vi "Prefilter.60Hz_Notch.vi"(8 "error in (no error)":errorcluster, 11 "Instrument.DAQ":refnum<class "Instrument.DAQ.lvclass">) -> (0 "error out":errorcluster, 3 "Instrument.DAQ out":refnum<class "Instrument.DAQ.lvclass">)   [LabVIEW 2019, in "Instrument.Lockin.lvlib" / "Instrument.DAQ.lvclass"]
uses:
  Instrument.DAQ.lvclass
  Instrument.DAQ.lvclass/Instrument.DAQ.ctl
  <vilib>/addons/Digital Filter Design/Design.llb/DFD IIR Notch Peak Design by Q.vi
  <vilib>/addons/Digital Filter Design/NI_DigFilterLicensed.lvlib
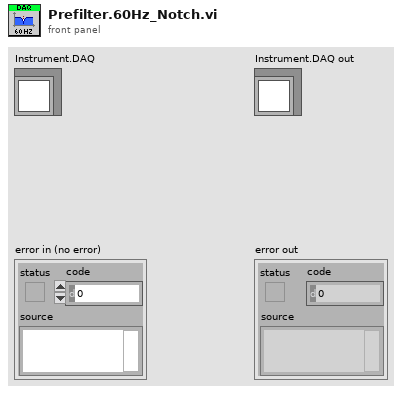
[diagram p1: front panel]
types:
  T1 = typedef "NI_DigFilterLicensed.lvlib/DFD Filter Obj.ctl" = cluster{"mSRate_Fs":dbl, "mSRate_Version":string, "mSRate_Comments":string, "mSRate_OrgCoef":T2, "mSRate_CurCoef":T2, "mSRate_Quantized?":bool, "mSRate_QCoef":T2, "mSRate_QSettings":T4[], "mSRate_Order":i32, "mSRate_Scaling":cluster{"mSRate_ScaleByPowerOf2?":bool, "mSRate_ScaleType":T6}}
  T2 = typedef "NI_DigFilterLicensed.lvlib/DFD Filter Coef.ctl" = cluster{"type":T3, "gain":dbl, "coef a (k)":dbl[], "coef b (v)":dbl[]}
  T3 = typedef "NI_DigFilterLicensed.lvlib/DFD Filter Structure Type Selector.ctl" = enum16{"Undefined", "FIR Direct Form", "FIR Direct Form Transposed", "FIR Symmetric", "FIR Antisymmetric", "IIR Direct Form I", "IIR Direct Form I Transposed", "IIR Direct Form II", "IIR Direct Form II Transposed", "IIR Cascaded Second Order Sections Form I", "IIR Cascaded Second Order Sections Form I Transposed", "IIR Cascaded Second Order Sections Form II", "IIR Cascaded Second Order Sections Form II Transposed", "Lattice Allpass (basic sections)", "Lattice Allpass (one multiplier sections)", "Lattice Allpass (normalized sections)", "Lattice AR (basic sections)", "Lattice AR (one multiplier sections)", "Lattice AR (normalized sections)", "Lattice MA (minimum phase)", "Lattice MA (maximum phase)", "Lattice ARMA (basic sections)", "Lattice ARMA (one multiplier sections)", "Lattice ARMA (normalized sections)"}
  T4 = typedef "NI_DigFilterLicensed.lvlib/dfd_Internal Quantization Settings.ctl" = cluster{"source":T5, "wl":i16, "iwl":i16, "overflow mode":enum16{"Saturation", "Wrap"}, "rounding mode":enum16{"Nearest", "Truncation"}, "signed?":bool}
  T5 = typedef "NI_DigFilterLicensed.lvlib/dfd_Internal Quantization Srcs.ctl" = u16
  T6 = typedef "NI_DigFilterLicensed.lvlib/DFD Coef Norm Type.ctl" = enum16{"No Norm", "Time Domain 1-Norm", "Time Domain 2-Norm", "Time Domain Inf-Norm"}
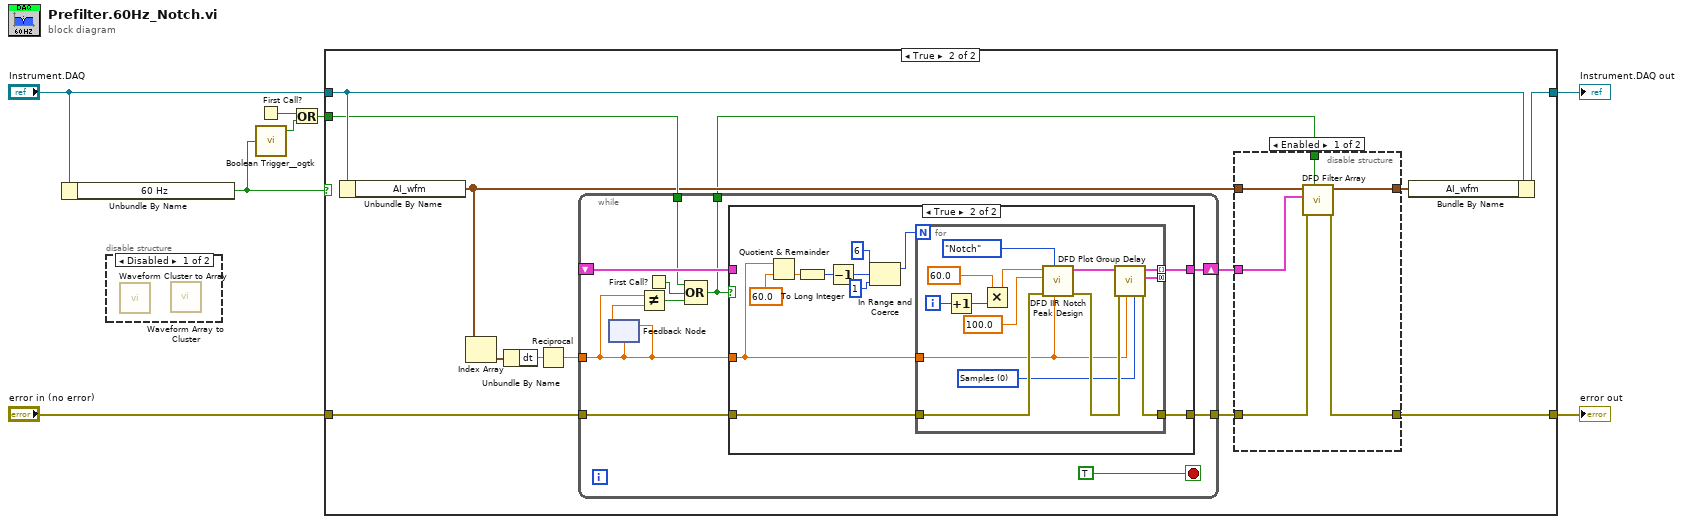
[diagram p0: block diagram]
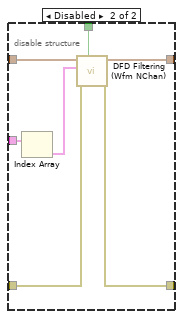
[diagram p5: hidden frame]
diagram:
  n1 = Unbundle By Name("Instrument.DAQ") -> ("60 Hz"=w2:bool)
  n2 = disable-structure shown="Disabled" {
    frame Disabled {
      n3 = call "Waveform Cluster to Array.vi"() -> ()  [unwired: 10 in, 2 out]
      n4 = call "Waveform Array to Cluster.vi"() -> ()  [unwired: 11 in, 1 out]
    }
    frame Enabled {
    }
  }
  n5 = First Call?() -> (First Call?: T/F=w4:bool)
  n6 = call <userlib>:"Boolean Trigger__ogtk.vi"("Boolean Input"=w2) -> ("Rising Edge"=w1:bool)  [unwired: 1 in, 1 out]
  n7 = Or(x=w4, y=w1) -> (x .or. y?=w3:bool)
  n8 = case shown="True" w2 {
    tunnel: "error in (no error)" -> [w9 w23]
    tunnel: [w9 w17] -> w7
    tunnel: "Instrument.DAQ" -> [w10 w20]
    tunnel: [w10 w16] -> w6
    tunnel: w3 -> [_ w14]
    frame False {
    }
    frame True {
      n9 = Unbundle By Name(w20) -> ("AI_wfm"=w13:waveform(dbl)[])
      n10 = Index Array(array=w13) -> (element=w21:waveform(dbl))  [unwired: 1 in]
      n11 = Unbundle By Name(w21) -> ("dt"=w22:dbl)
      n12 = Reciprocal(x=w22) -> (1/x=w19:dbl)
      n13 = while {
        shift-right: [w33] -> w12
        shift-left: _ -> [w26]
        tunnel: w19 -> [w32]
        tunnel: w23 -> [w34]
        tunnel: [w27] -> w15
        tunnel: w14 -> [w25]
        tunnel: [w24] -> w11
        stop <- TRUE stop-if-true
        n14 = feedback #1(w32) -> (w31:dbl)
        n15 = feedback-in #1(w32) -> ()
        n16 = Not Equal?(x=w32, y=w31) -> (x != y?=w30:bool)
        n17 = First Call?() -> (First Call?: T/F=w29:bool)
        n18 = Compound Arithmetic op=OR(w25, w29, w30) -> (w24:bool)
        n19 = case shown="True" w24 {
          tunnel: w34 -> [w35 w47]
          tunnel: [w36 w45] -> w33
          tunnel: w32 -> [_ w46]
          tunnel: [w35 w44] -> w27
          tunnel: w26 -> [w36 _]
          frame False {
          }
          frame True {
            n20 = Quotient & Remainder(x=w46, y=60.0 ("f0 [Hz]")) -> (floor(x/y)=w42:dbl)  [unwired: 1 out]
            n21 = To Long Integer(number=w42) -> (32bit integer=w43:i32)
            n22 = Decrement(x=w43) -> (x-1=w40:i32)
            n23 = In Range and Coerce(upper limit=6, x=w40, lower limit=1) -> (coerced(x)=w37:i32)  [unwired: 1 out]
            n24 = for {
              N: w37 -> [_]
              tunnel: w46 -> [w48]
              tunnel: [w52] -> w45 mode=indexing
              tunnel: w47 -> [w61]
              tunnel: [w51] -> w44
              tunnel: [w49] -> _ mode=concatenating
              i -> [w56]
              w50 = u16 0 items=["Samples", "Seconds"] ("group delay unit")
              n25 = Increment(x=w56) -> (x+1=w58:i32)
              n26 = Multiply(x=60.0 ("f0 [Hz]"), y=w58) -> (x*y=w55:dbl)
              n27 = call-poly <vilib>:"DFD IIR Notch Peak Design.vi"("fs [Hz]"=w48, "filter type"=enum16{"Notch", "Peak"}."Notch", "error in (no error)"=w61, "Q factor"=100.0, "f0 [Hz]"=w55) -> ("error out"=w54:errorcluster, "filter out"=w53:T1)  [unwired: 5 in]
              n28 = call <vilib>:"DFD Plot Group Delay.vi"("group delay unit"=w50, "fs [Hz]"=w48, "error in (no error)"=w54, "filter in"=w53) -> ("error out"=w51:errorcluster, "group delay"=w49:cluster{"f0":dbl, "df":dbl, "values":dbl[]}[], "filter out"=w52:T1)  [unwired: 5 in]
            }
          }
        }
      }
      n29 = disable-structure shown="Enabled" {
        disable-tunnel: [w67 w73] -> w18
        disable-tunnel: [w66 w70] -> w17
        disable-tunnel: w15 -> [w65 w71]
        disable-tunnel: w13 -> [w64 w74]
        disable-tunnel: w12 -> [w63 w69]
        disable-tunnel: w11 -> [w62 w72]
        frame Enabled {
          n30 = call "DFD Filter Array.vi"("init (F)"=w62, "error in (no error)"=w65, "filters"=w63, "signal in"=w64) -> ("error out"=w66:errorcluster, "signal out"=w67:waveform(dbl)[])  [unwired: 6 in]
        }
        frame Disabled {
          n31 = Index Array(array=w69) -> (element=w68:T1)  [unwired: 1 in]
          n32 = call <vilib>:"DFD Filtering (Wfm NChan).vi"("init? (F)"=w72, "error in (no error)"=w71, "filter"=w68, "signal in"=w74) -> ("error out"=w70:errorcluster, "signal out"=w73:waveform(dbl)[])  [unwired: 6 in]
        }
      }
      n33 = Bundle By Name(cluster=w20, "AI_wfm"=w18) -> (w16:refnum<class "Instrument.DAQ.lvclass">)
    }
  }
  "error out" <- w7
  "Instrument.DAQ out" <- w6
